vi "ReadSweepMeasurement.vi"(8 "error in (no error)":errorcluster, 11 "9770 API in":refnum<class "9770 API.lvclass">) -> (0 "error out":errorcluster, 1 "sweep valid":bool, 2 "sweep":cluster{"frequency":dbl, "amplitude":dbl}[](array[cluster]), 3 "9770 API out":refnum<class "9770 API.lvclass">, 4 "sweep time (seconds)":dbl, 5 "ChannelName":string, 6 "current sweep frequency":dbl, 7 "Units":string)   [LabVIEW 2017, in "9770 API.lvclass"]
uses:
  <vilib>/addons/InsightCM/Devices/Shared/Emsa/Emsa9770API/9770 API.lvclass
  <vilib>/addons/InsightCM/Devices/Shared/Emsa/Emsa9770API/9770 API.lvclass/9770 API.ctl
panel:
  out "samples remaining":u32
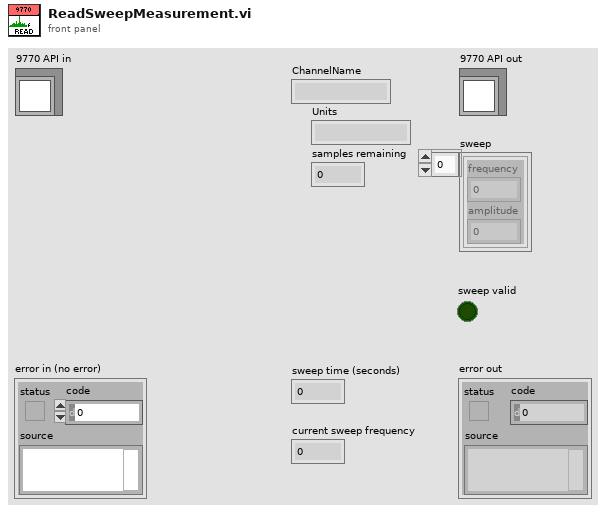
[diagram p1: front panel]
types:
  T1 = cluster{"Sweep":cluster{"Center Freq":dbl, "Bandwidth":dbl}[], "SampleRate":dbl, "FullScaleVoltage":dbl, "DetectionTime":dbl, "DetectionMode":enum16{"Peak", "Quasi Peak", "Average"}}
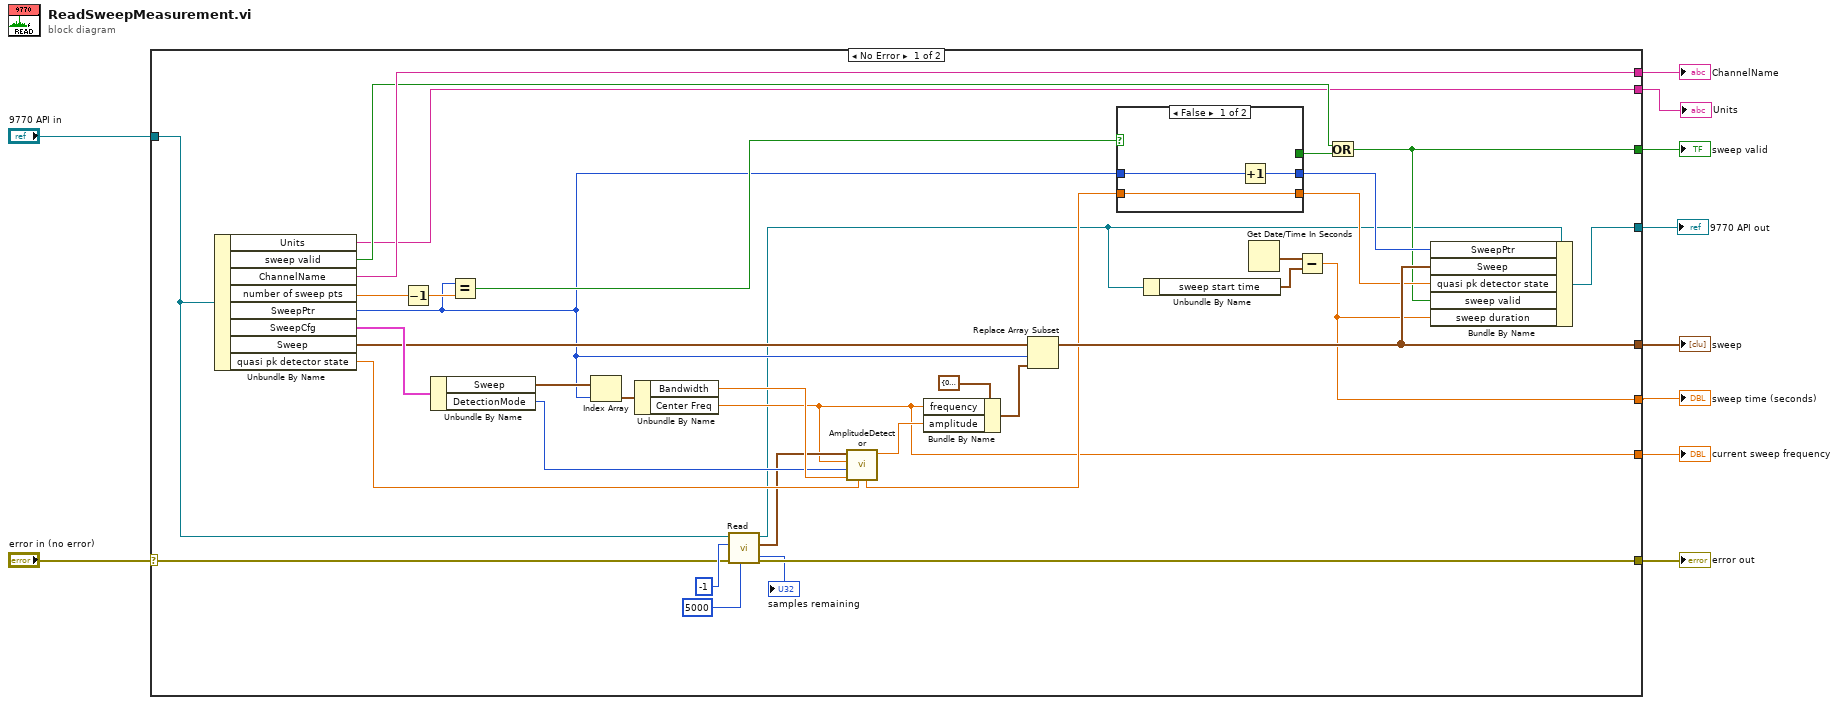
[diagram p0: block diagram]
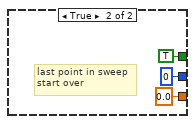
[diagram p2: hidden frame]
diagram:
  n1 = case shown="No Error" "error in (no error)" {
    selector: "error in (no error)" -> [w13 w54]
    tunnel: [w31 w54] -> w9
    tunnel: [w27 w53] -> w7
    tunnel: "9770 API in" -> [w12 w53]
    tunnel: [w22 _] -> w6
    tunnel: [w32 _] -> w5
    tunnel: [w25 _] -> w4
    tunnel: [w16 _] -> w3
    tunnel: [w19 _] -> w2
    tunnel: [w14 _] -> w1
    frame No Error {
      n2 = Unbundle By Name(w12) -> ("Units"=w14:string, "sweep valid"=w21:bool, "ChannelName"=w25:string, "number of sweep pts"=w38:dbl, "SweepPtr"=w24:i32, "SweepCfg"=w46:T1, "Sweep"=w36:cluster{"frequency":dbl, "amplitude":dbl}[], "quasi pk detector state"=w30:dbl)
      n3 = Decrement(x=w38) -> (x-1=w37:dbl)
      n4 = Unbundle By Name(w46) -> ("Sweep"=w45:cluster{"Center Freq":dbl, "Bandwidth":dbl}[], "DetectionMode"=w39:enum16{"Peak", "Quasi Peak", "Average"})
      n5 = Equal?(x=w24, y=w37) -> (x = y?=w33:bool)
      n6 = Index Array(array=w45, index=w24) -> (element=w44:cluster{"Center Freq":dbl, "Bandwidth":dbl})
      n7 = Unbundle By Name(w44) -> ("Bandwidth"=w40:dbl, "Center Freq"=w19:dbl)
      n8 = call <vilib>:"Read.vi"("timeout (ms)"=5000, "error in (no error)"=w13, "number of samples"=-1, "9770 API in"=w12) -> ("error out"=w31:errorcluster, "Waveform"=w20:waveform(cdb), "9770 API out"=w15:refnum<class "9770 API.lvclass">, "samples remaining"=→"samples remaining":u32)  [unwired: 2 in, 2 out]
      n9 = call <vilib>:"AmplitudeDetector.vi"("quasi peak detector in"=w30, "resolution bandwidth"=w40, "DetectionMode"=w39, "frequency"=w19, "waveform"=w20) -> ("Value"=w26:dbl, "quasi peak detector out"=w29:dbl)  [unwired: 4 in, 1 out]
      n10 = Bundle By Name(cluster=cluster{"frequency":dbl, "amplitude":dbl} {"frequency"=0.0, "amplitude"=0.0} ("new element/subarray"), "frequency"=w19, "amplitude"=w26) -> (w34:cluster{"frequency":dbl, "amplitude":dbl})
      n11 = Replace Array Subset(array=w36, new element=w34, index=w24) -> (w32:cluster{"frequency":dbl, "amplitude":dbl}[])
      n12 = case shown="False" w33 {
        tunnel: [w49 0] -> w41
        tunnel: w24 -> [w48 _]
        tunnel: w29 -> [w47 _]
        tunnel: [w47 0.0 ("quasi peak detector out")] -> w28
        tunnel: [_ TRUE] -> w23
        frame False {
          n13 = Increment(x=w48) -> (x+1=w49:i32)
        }
        frame True {
          # "last point in sweep\nstart over"
        }
      }
      n14 = Unbundle By Name(w15) -> ("sweep start time"=w18:timestamp)
      n15 = Get Date/Time In Seconds() -> (seconds since 1Jan1904=w17:timestamp)
      n16 = Subtract(x=w17, y=w18) -> (x-y=w16:dbl)
      n17 = Or(x=w21, y=w23) -> (x .or. y?=w22:bool)
      n18 = Bundle By Name(cluster=w15, "SweepPtr"=w41, "Sweep"=w32, "quasi pk detector state"=w28, "sweep valid"=w22, "sweep duration"=w16) -> (w27:refnum<class "9770 API.lvclass">)
    }
    frame Error {
    }
  }
  "error out" <- w9
  "9770 API out" <- w7
  "sweep valid" <- w6
  "sweep" <- w5
  "ChannelName" <- w4
  "sweep time (seconds)" <- w3
  "current sweep frequency" <- w2
  "Units" <- w1
